vi "MSGError.vi"(8 "error in (no error)":errorcluster, 11 "IncomingString":string) -> (0 "error out":errorcluster, 3 "OutputString":string)   [LabVIEW 2023]
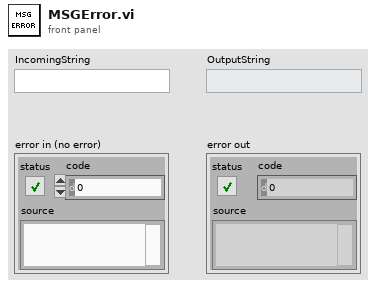
[diagram p1: front panel]
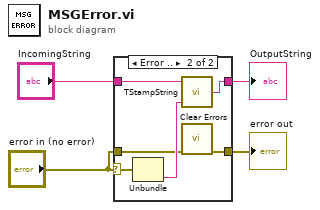
[diagram p0: block diagram]
diagram:
  n1 = case shown="Error .." "error in (no error)" {
    selector: "error in (no error)" -> [_ w12]
    tunnel: "error in (no error)" -> [w6 w10]
    tunnel: [w6 w9] -> w4
    tunnel: "IncomingString" -> [w5 w8]
    tunnel: [w5 w7] -> w2
    frame No Error {
    }
    frame Error {
      n2 = Unbundle(w12) -> ("source"=w11:string)  [unwired: 2 out]
      n3 = call "TStampString.vi"("Incoming string"=w11, "Previous string"=w8) -> ("String with time stamp"=w7:string)  [unwired: 1 in]
      n4 = call <vilib>:"Clear Errors.vi"("error in (no error)"=w10) -> ("error out"=w9:errorcluster)  [unwired: 5 in, 1 out]
    }
  }
  "error out" <- w4
  "OutputString" <- w2
